vi "Image Destination.vi"(1 "Images Destination In":path=path "") -> (0 "Images Destination Out":path)   [LabVIEW 2018, in "Scripts.lvlib"]
uses:
  Scripts.lvlib
  <vilib>/Field R&D Services/Labricator/Toolkit/Labricator.lvlib
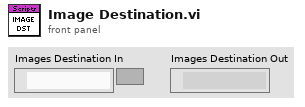
[diagram p1: front panel]
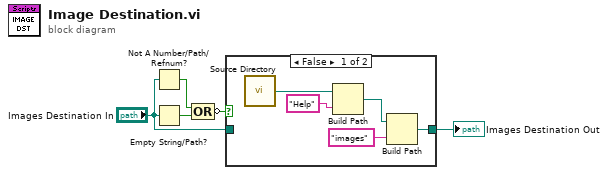
[diagram p0: block diagram]
diagram:
  n1 = Not A Number/Path/Refnum?(number/path/refnum="Images Destination In") -> (NaN/Path/Refnum?=w2:bool)
  n2 = Empty String/Path?(string/path="Images Destination In") -> (empty?=w1:bool)
  n3 = Compound Arithmetic op=OR(w2, w1) -> (invert w3:bool)
  n4 = case shown="False" w3 {
    tunnel: "Images Destination In" -> [_ w11]
    tunnel: [w6 w11] -> w5
    frame False {
      n5 = call <vilib>:"Source Directory.vi"() -> ("Source Directory"=w10:path)
      n6 = Build Path(base path=w10, name or relative path="Help") -> (appended path=w8:path)
      n7 = Build Path(base path=w8, name or relative path="images") -> (appended path=w6:path)
    }
    frame True {
    }
  }
  "Images Destination Out" <- w5
